vi "combination.vi"(8 "b":i32, 11 "a":i32) -> (2 "ans":i64)   [LabVIEW 2023]
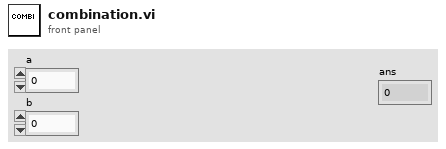
[diagram p1: front panel]
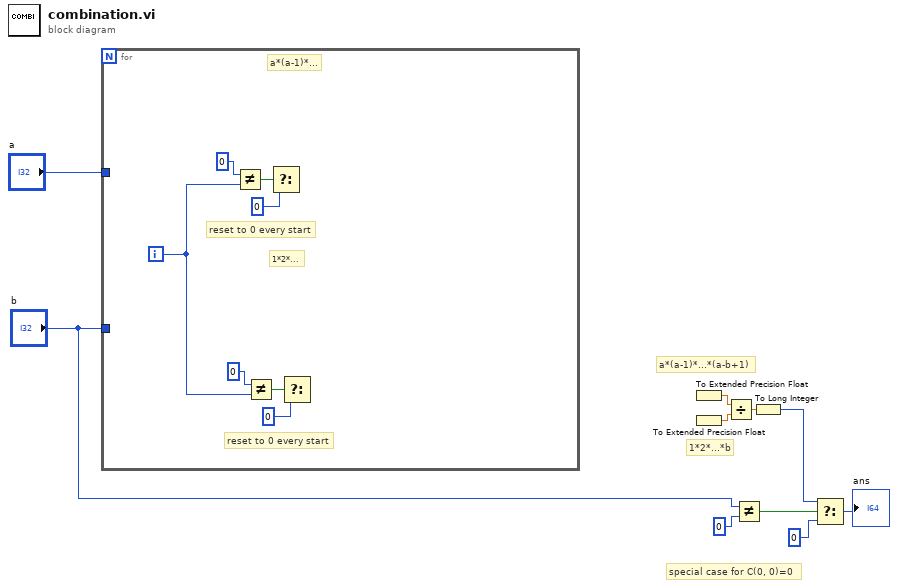
[diagram p0: block diagram]
diagram:
  # "1*2*...*b"
  # "a*(a-1)*...*(a-b+1)"
  # "special case for C(0, 0)=0"
  n1 = for {
    tunnel: "a" -> [_]
    tunnel: "b" -> [_]
    i -> [w11]
    # "1*2*..."
    # "a*(a-1)*..."
    # "reset to 0 every start"
    # "reset to 0 every start"
    n2 = Not Equal?(x=0, y=w11) -> (x != y?=w16:bool)
    n3 = Not Equal?(x=0, y=w11) -> (x != y?=w13:bool)
    n4 = Select(s=w16, f=0 ("x")) -> ()  [unwired: 1 in, 1 out]
    n5 = Select(s=w13, f=0 ("x")) -> ()  [unwired: 1 in, 1 out]
  }
  n6 = To Extended Precision Float() -> (0:w7:ext)  [unwired: 1 in]
  n7 = To Extended Precision Float() -> (0:w6:ext)  [unwired: 1 in]
  n8 = Divide(x=w7, y=w6) -> (x/y=w2:ext)
  n9 = Not Equal?(x="b", y=0) -> (x != y?=w9:bool)
  n10 = To Long Integer(number=w2) -> (32bit integer=w1:i32)
  n11 = Select(t=w1, s=w9, f=i64 0) -> (s? t:f=→"ans":i64)
